vi "Obtain MHL Queue.vi"(8 "ErrorIn":errorcluster, 11 "Create New (F)":bool) -> (0 "ErrorOut":errorcluster, 3 "MHL Queue Out":refnum<queue>)   [LabVIEW 2020, in "main.lvlib"]
doc: "Obtain Queue"
uses:
  main.lvlib
  PTRL/dev_and_debug_tools/QueueMessage typedef.ctl
  PTRL/QueueHandler/SubVis/Initialise.vi
  PTRL/QueueHandler/QueueHandler.lvlib
  PTRL/dev_and_debug_tools/dev_and_debug_tools.lvlib
panel:
  # "Description\n\nObtain Queue"
  # "INPUTS"
  # "OUTPUTS"
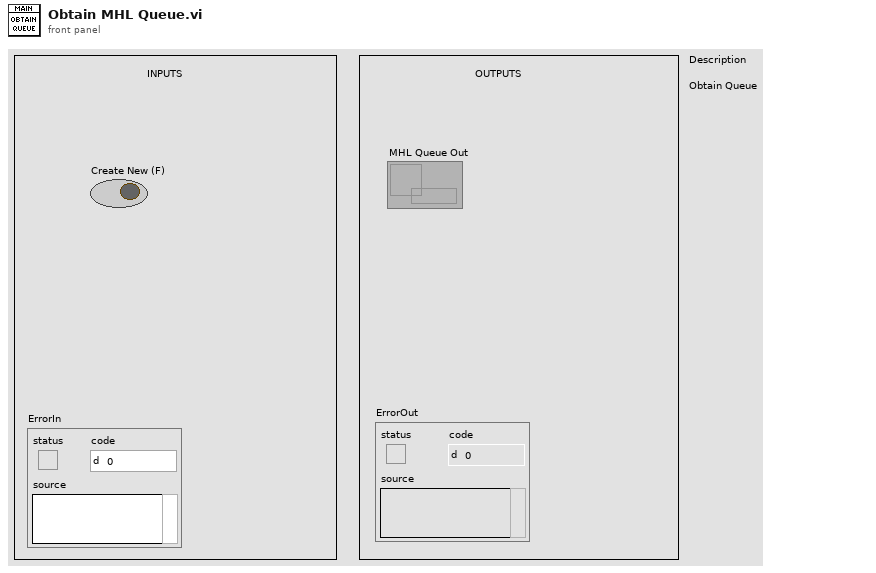
[diagram p1: front panel]
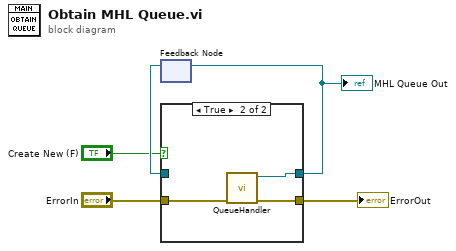
[diagram p0: block diagram]
diagram:
  n1 = feedback #1() -> (w4:refnum<queue>)  [unwired: 1 in]
  n2 = case shown="True" "Create New (F)" {
    tunnel: w4 -> [w7 _]
    tunnel: [w7 w8] -> w5
    tunnel: [w6 w10] -> w1
    tunnel: "ErrorIn" -> [w6 w9]
    frame False {
    }
    frame True {
      n3 = call-poly "QueueHandler.vi"("ErrorIn"=w9) -> ("ErrorOut"=w10:errorcluster, "queue out"=w8:refnum<queue>)  [unwired: 8 in, 1 out]
    }
  }
  "ErrorOut" <- w1
  "MHL Queue Out" <- w5
  n4 = feedback-in #1(w5) -> ()
